vi "Parse BTI MSGACT.vi"(11 "msgact":u16 format="%016b") -> (0 "specific errors":T1, 1 "receiving error":bool, 2 "hit":bool, 3 "hardware channel":u8, 4 "speed":enum16{"Low", "High"}(ring))   [LabVIEW 2020, in "AIM ARINC 429 Engine.lvlib" / "Custom Device.lvlib"]
uses:
  Custom Device.lvlib
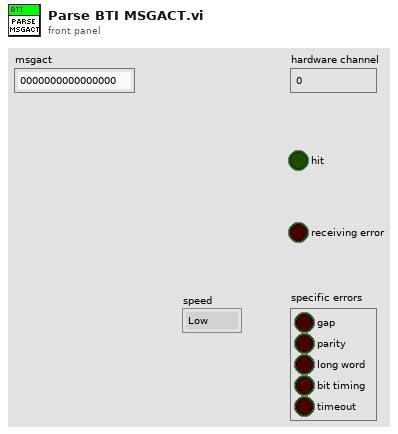
[diagram p1: front panel]
types:
  T1 = cluster{"gap":bool, "parity":bool, "long word":bool, "bit timing":bool, "timeout":bool}
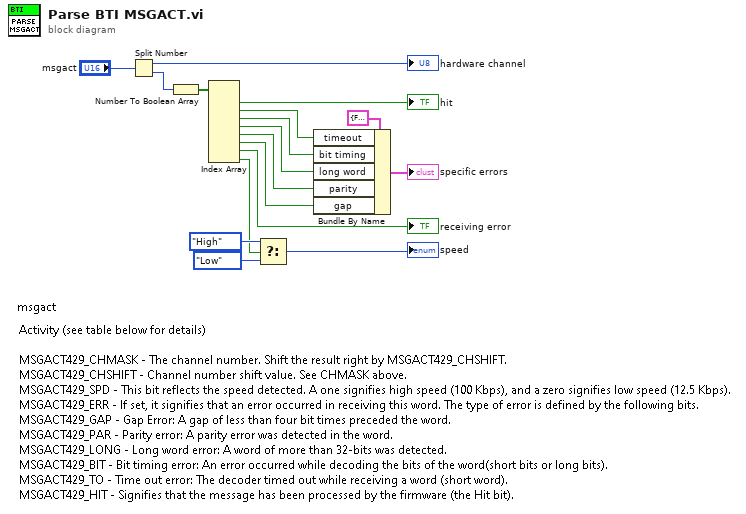
[diagram p0: block diagram]
diagram:
  n1 = Split Number(x="msgact") -> (hi(x)=→"hardware channel":u8, lo(x)=w15:u8)
  n2 = Number To Boolean Array(number=w15) -> (Boolean array=w14:bool[])
  n3 = Index Array(array=w14) -> (element #1=→"hit":bool, element #2=w6:bool, element #3=w5:bool, element #4=w4:bool, element #5=w3:bool, element #6=w2:bool, element #7=→"receiving error":bool, element #8=w9:bool)  [unwired: 8 in]
  n4 = Select(t=enum16{"Low", "High"}."High" ("speed"), s=w9, f=enum16{"Low", "High"}."Low" ("speed")) -> (s? t:f=→"speed":enum16{"Low", "High"})
  n5 = Bundle By Name(cluster=T1 {"gap"=FALSE, "parity"=FALSE, "long word"=FALSE, "bit timing"=FALSE, "timeout"=FALSE} ("specific errors"), "timeout"=w6, "bit timing"=w5, "long word"=w4, "parity"=w3, "gap"=w2) -> (→"specific errors":T1)
